vi "TestSpeed.vi"() -> ()   [LabVIEW 2016, in "Moving Motor.lvrbt"]
uses:
  Moving Motor.lvrbt
  <vilib>/NXT/Hardware/Plugins/Tetrix DC Motor/TetrixDCMotorAddress.ctl
  <vilib>/NXT/NXTIO Xnodes/NXTIONodeSubVIs/TETRIX IO Move DC Motors.vi
  <vilib>/NXT/Subs/LVHSConnector.ctl
  <vilib>/NXT/NXTIO Xnodes/AddressXNode/NXTIOAddress.xnode
  <vilib>/NXT/NXTIO Xnodes/NXTIOXNode/NXTIO.xnode
  <vilib>/NXT/LegoClasses/BrickReference/BrickReference.lvclass
panel:
  in  "stop":bool
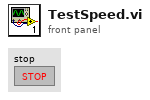
[diagram p1: front panel]
types:
  T1 = typedef "TetrixDCMotorAddress.ctl" = i32
  T2 = cluster{"TetrixDCMotor":T1, "TetrixDCMotor 2":T1}
  T3 = typedef "LVHSConnector.ctl" = refnum<class "BrickReference.lvclass">
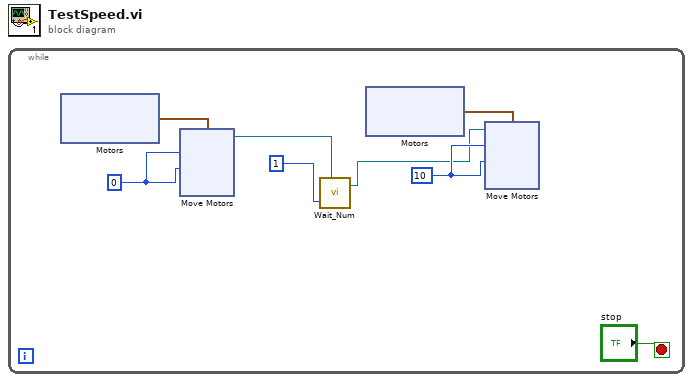
[diagram p0: block diagram]
diagram:
  n1 = while {
    stop <- "stop" stop-if-true
    w2 = 10
    w7 = 0
    n2 = xnode "Motors"() -> ("Motor"=w8:cluster{"TetrixDCMotor":T1, "TetrixDCMotor":T1})
    n3 = xnode "Move Motors"("Power/Speed 2"=w7, "Power/Speed 1"=w7, "Motors"=w8) -> ("NXT/EV3"=w5:T3)  [unwired: 1 in]
    n4 = call <vilib>:"Wait_Num.vi"("Time (1 sec)"=1, "NXT/EV3"=w5) -> ("NXT/EV3"=w1:T3)  [unwired: 2 in]
    n5 = xnode "Motors"() -> ("Motor"=w3:cluster{"TetrixDCMotor":T1, "TetrixDCMotor":T1})
    n6 = xnode "Move Motors"("Power/Speed 2"=w2, "Power/Speed 1"=w2, "Motors"=w3, "NXT/EV3"=w1) -> ()  [unwired: 1 out]
  }
